vi "Modbus Comm Tester.vi"() -> ()   [LabVIEW 2012]
doc: "Modbus Comm Tester\n\nThis VI demonstrates the usage of the Modbus Master API for both TCP and Serial connections.\nIt is also a useful tool for testing communication with your modbus device. You can test different\ncommunication parameters and coil/register address ranges without having to write any code.\n\nCopyright (c) 2016, Plasmionique Inc.\nAll rights reserved.\n\nLicense: BSD (2-Clause) - http://opensource.org/licenses/BSD-2-Clause"
uses:
  MB_PDU/MB_ReadDevID Codes.ctl
  MB_Master/MB_Master.lvclass
  MB_Master_TCP/MB_Master_TCP.lvclass
  MB_ADU/MB_ADU.lvclass/MB_ADU.ctl
  MB_ADU/Read TX Data.vi
  MB_ADU/Read RX Data.vi
  MB_ADU/Read RX Timestamp.vi
  MB_Master_Serial/MB_Master_Serial.lvclass
  MB Master.lvlib
  MB_ADU/MB_ADU.lvclass
panel:
  in  "Device ID code":T1=1 items=["Basic"=1, "Regular"=2, "Extended"=3, "Single"=4]
  in  "object ID":u8 caption="Object ID"
  in  "Read ID":bool
  out "Open?":bool caption="Connected"
  in  "Tab Control 2":enum32{"Comm Settings", "Comm Status"}(tab)
  in  "Open":bool
  in  "Close":bool
  in  "Type":enum16{"Serial", "TCP"}(ring) caption="Connection Type"
  in  "Tab Control":enum32{"Page 1", "Page 2"}(tab)
  in  "Retries":i32=1
  in  "Timeout (ms)":u32=300
  in  "Flow Control":u16(ring) items=["None", "XON/XOFF", "RTS/CTS", "XON/XOFF & RTS/CTS", "DTR/DSR", "XON/XOFF & DTR/DSR"]
  in  "Parity":u16(ring) items=["None", "Odd", "Even", "Mark", "Space"]
  in  "Stop Bits":u16(ring)=10 items=["1.0"=10, "1.5"=15, "2.0"=20]
  in  "Baud Rate (bps)":u32(ring)=19200 items=["9600"=9600, "19200"=19200, "38400"=38400, "57600"=57600, "115200"=115200, "460800"=460800, "921600"=921600]
  in  "Slave Address":u8=1
  in  "Mode":enum16{"RTU", "ASCII"}(ring)
  in  "COM Port":refnum<visa-resource-name>
  in  "TCP_Port":u16=502 caption="Port"
  in  "IP Address":string="localhost"
  in  "TCP_Timeout":i32=10000 caption="Timeout (ms)"
  in  "TCP_Slave ID":u8=255 caption="Slave ID" format="%.0x"
  in  "Poll Period (ms)":i32=100
  out "Last Error Status":errorcluster
  out "Last RX":string
  out "Last TX":string
  out "Last RX Time":string
  out "Last Error Time":string
  out "dt (ms)":u32
  out "ID objects":string[](array[string]) caption="ID Objects"
  in  "coil Poll":bool
  in  "HR Poll":bool
  in  "DI Poll":bool
  in  "IR Poll":bool
  in  "Write Hld Regs":bool
  in  "Read Hld Regs":bool
  in  "HR QTY":u16=1 caption="Quantity"
  in  "HR SA":u16 caption="Starting Address" format="%.0x"
  in  "Holding Registers":u16[](array[numeric])
  in  "Read In Regs":bool
  in  "IR QTY":u16=1 caption="Quantity"
  in  "IR SA":u16 caption="Starting Address" format="%.0x"
  out "Input Registers":u16[](array[numeric])
  in  "Read DIs":bool
  in  "DI QTY":u16=1 caption="Quantity"
  in  "DI SA":u16 caption="Starting Address" format="%.0x"
  out "Discrete Inputs":bool[](array[boolean])
  in  "Write Coils":bool
  in  "Read Coils":bool
  in  "Coil QTY":u16=1 caption="Quantity"
  in  "Coil SA":u16 caption="Starting Address" format="%.0x"
  in  "Coils":bool[](array[boolean])
  # "Input Registers"
  # "Discrete Inputs"
  # "Device ID Objects"
  # "Holding Registers"
  # "Coils"
  # "Communication Settngs"
  # "Communication Status"
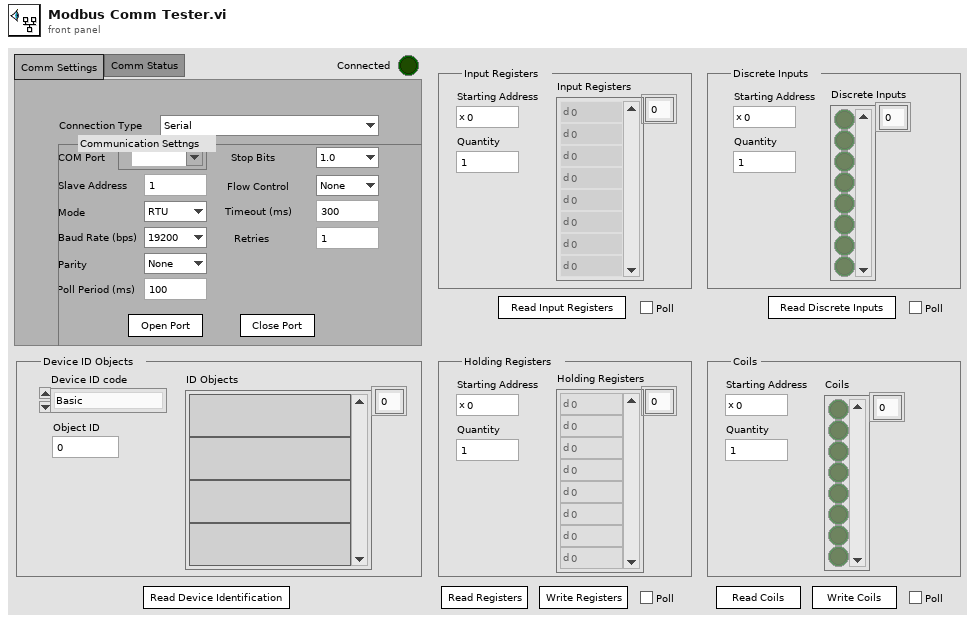
[diagram p1: front panel]
types:
  T1 = typedef "MB Master.lvlib/MB_ReadDevID Codes.ctl" = u8
  T2 = cluster{"baud rate (bps)":u32, "stop bits":u16, "parity":u16, "flow control":u16, "timeout":u32, "retries":i32}
  T3 = typedef "MB Master.lvlib/MB_DevID Object.ctl" = cluster{"ID":u8, "Value":string}
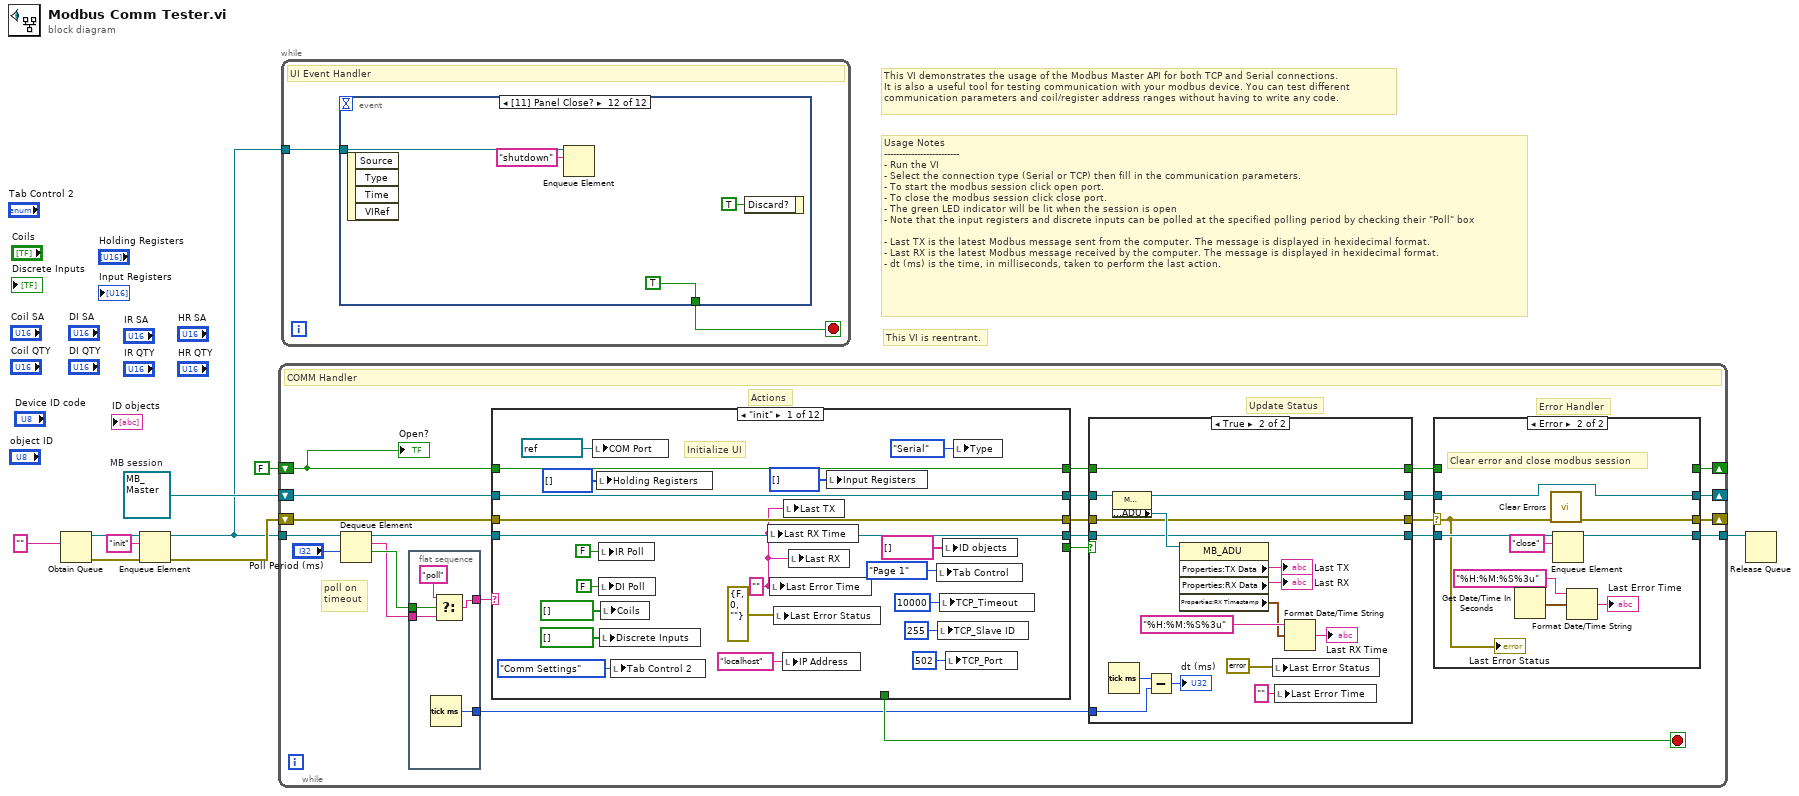
[diagram p0: block diagram]
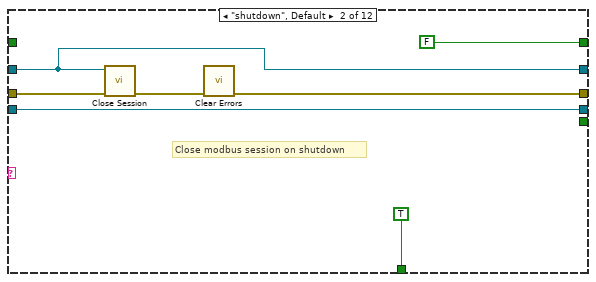
[diagram p4: hidden frame]
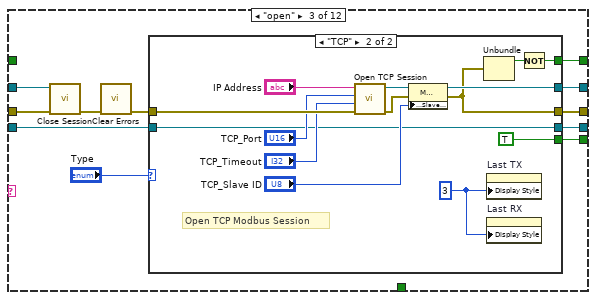
[diagram p5: hidden frame]
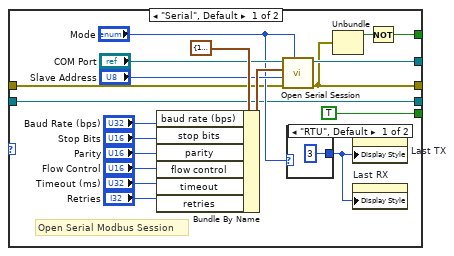
[diagram p6: hidden frame]
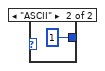
[diagram p7: hidden frame]
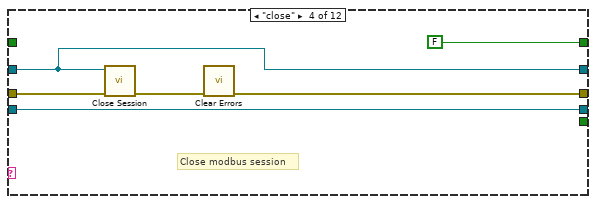
[diagram p8: hidden frame]
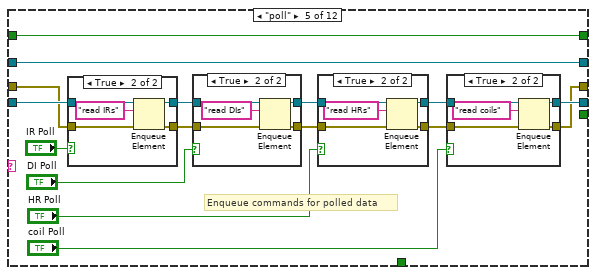
[diagram p9: hidden frame]
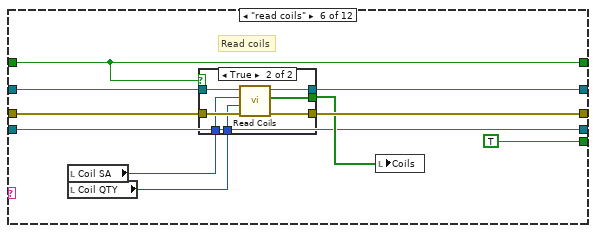
[diagram p14: hidden frame]
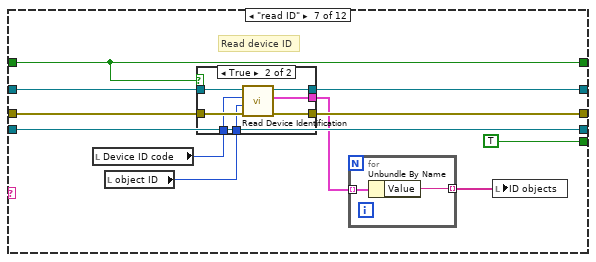
[diagram p16: hidden frame]
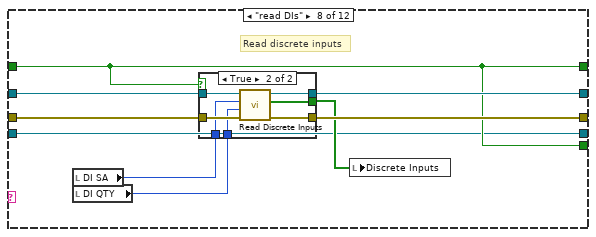
[diagram p18: hidden frame]
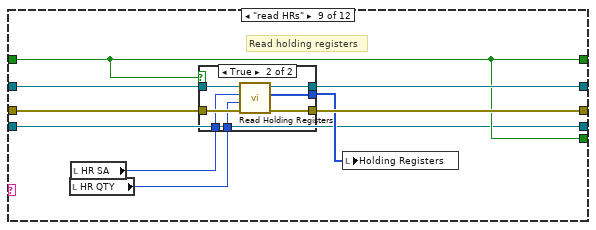
[diagram p20: hidden frame]
diagram:
  w7 = refnum<class "MB_Master.lvclass"> refnum  # MB session
  # "This VI is reentrant."
  # "Usage Notes\n-------------------------\n- Run the VI\n- Select the connection type (Serial or TCP) then fill in the communication parameters.\n- To start the modbus session click open port.\n- To close the modbus session click close port.\n- The green LED indicator will be lit when the session is open\n- Note that the input registers and discrete inputs can be polled at the specified polling period by checking their \"Poll\" box\n\n- Last TX is the latest Modbus message sent from the computer. The message is displayed in hexidecimal format.\n- Last RX is the latest Modbus message received by the computer. The message is displayed in hexidecimal format. \n- dt (ms) is the time, in milliseconds, taken to perform the last action."
  # "This VI demonstrates the usage of the Modbus Master API for both TCP and Serial connections.\nIt is also a useful tool for testing communication with your modbus device. You can test different\ncommunication parameters and coil/register address ranges without having to write any code."
  n1 = Obtain Queue(element data type="") -> (queue out=w6:refnum<queue>, error out=w4:errorcluster)  [unwired: 4 in, 1 out]
  n2 = Enqueue Element(queue=w6, element="init", error in (no error)=w4) -> (queue out=w2:refnum<queue>, error out=w3:errorcluster)  [unwired: 1 in, 1 out]
  n3 = while {
    tunnel: w2 -> [w33]
    shift-right: [w16] -> _
    shift-left: w7 -> [w32]
    shift-right: [w23] -> _
    shift-left: w3 -> [w24]
    shift-right: [w18] -> _
    shift-left: FALSE -> [w28]
    tunnel: [w22] -> w1
    stop <- w31 stop-if-true
    # "poll on\ntimeout"
    # "Actions"
    # "Error Handler"
    # "Update Status"
    # "COMM Handler"
    n4 = Dequeue Element(queue=w33, timeout in ms (-1)="Poll Period (ms)") -> (queue out=w30:refnum<queue>, element=w20:string, timed out?=w21:bool)  [unwired: 1 in, 1 out]
    n5 = flat-sequence {
      tunnel: [w51] -> w25
      tunnel: w21 -> [w50]
      tunnel: w20 -> [w49]
      tunnel: [w47] -> w19
      frame #0 {
        n6 = Tick Count (ms)() -> (millisecond timer value=w51:u32)
        n7 = Select(t="poll", s=w50, f=w49) -> (s? t:f=w47:string)
      }
    }
    n8 = case shown="\"init\"" w19 {
      tunnel: [w91 w96 w110 w148 w160 w203 w223 w243 w261 w279 w299 w333] -> w29
      tunnel: w32 -> [w91 w96 w105 w148 w160 w205 w225 w245 w263 w281 w302 w336]
      tunnel: [w90 w97 w109 w149 w152 w202 w222 w242 w260 w278 w297 w331] -> w13
      tunnel: w24 -> [w90 w99 w104 w151 w164 w204 w224 w244 w262 w280 w298 w332]
      tunnel: [_ TRUE _ _ _ _ _ _ _ _ _ _] -> w31
      tunnel: w30 -> [w81 w93 w101 w146 w166 w196 w219 w237 w255 w273 w291 w325]
      tunnel: w28 -> [w88 _ _ _ w161 w200 w221 w238 w256 w274 w292 w326]
      tunnel: [w88 FALSE w108 FALSE w161 w200 w221 w238 w256 w274 w292 w326] -> w15
      tunnel: [_ _ w107 _ _ TRUE TRUE w238 w256 w274 w292 w326] -> w27
      tunnel: [w81 w93 w100 w146 w158 w196 w219 w237 w255 w273 w291 w325] -> w11
      frame "init" {
        w89 = "" ("Last Error Time")
        # "Initialize UI"
        n9 = local write "COM Port"(refnum<visa-resource-name> refnum ("COM Port")) -> ()
        n10 = local write "Holding Registers"(u16[] [] ("Holding Registers")) -> ()
        n11 = local write "IR Poll"(FALSE ("IR Poll")) -> ()
        n12 = local write "DI Poll"(FALSE ("DI Poll")) -> ()
        n13 = local write "Discrete Inputs"(bool[] [] ("Coils")) -> ()
        n14 = local write "Coils"(bool[] [] ("Coils")) -> ()
        n15 = local write "Tab Control 2"(enum32{"Comm Settings", "Comm Status"}."Comm Settings" ("Tab Control 2")) -> ()
        n16 = local write "Last RX Time"(w89) -> ()
        n17 = local write "Last Error Time"(w89) -> ()
        n18 = local write "Last Error Status"(errorcluster {"status"=FALSE, "code"=0, "source"=""} ("Last Error Status")) -> ()
        n19 = local write "IP Address"("localhost" ("IP Address")) -> ()
        n20 = local write "Last TX"(w89) -> ()
        n21 = local write "Last RX"(w89) -> ()
        n22 = local write "Input Registers"(u16[] [] ("Input Registers")) -> ()
        n23 = local write "Tab Control"(enum32{"Page 1", "Page 2"}."Page 1" ("Tab Control")) -> ()
        n24 = local write "TCP_Slave ID"(u8 255 ("TCP_Slave ID")) -> ()
        n25 = local write "TCP_Timeout"(10000 ("TCP_Timeout")) -> ()
        n26 = local write "ID objects"(string[] [] ("ID objects")) -> ()
        n27 = local write "TCP_Port"(u16 502 ("TCP_Port")) -> ()
        n28 = local write "Type"(enum16{"Serial", "TCP"}."Serial" ("Type")) -> ()
      }
      frame "shutdown", Default {
        # "Close modbus session on shutdown"
        n29 = call-dynamic "Close Session.vi"("error in (no error)"=w99, "MB session in"=w96) -> ("error out"=w98:errorcluster)  [unwired: 9 in]
        n30 = call <vilib>:"Clear Errors.vi"("error in (no error)"=w98) -> ("error out"=w97:errorcluster)  [unwired: 6 in]
      }
      frame "open" {
        n31 = call-dynamic "Close Session.vi"("error in (no error)"=w104, "MB session in"=w105) -> ("error out"=w106:errorcluster)  [unwired: 9 in]
        n32 = call <vilib>:"Clear Errors.vi"("error in (no error)"=w106) -> ("error out"=w103:errorcluster)  [unwired: 6 in]
        n33 = case shown="\"TCP\"" "Type" {
          tunnel: [w119 w136] -> w110
          tunnel: [w118 w134] -> w109
          tunnel: [w116 w133] -> w108
          tunnel: [TRUE TRUE] -> w107
          tunnel: w103 -> [w112 w143]
          tunnel: [w111 w137] -> w100
          tunnel: w101 -> [w111 w137]
          frame "Serial", Default {
            # "Open Serial Modbus Session"
            n34 = Bundle By Name(cluster=T2 {"baud rate (bps)"=19200, "stop bits"=10, "parity"=0, "flow control"=0, "timeout"=1000, "retries"=1} ("Serial Config"), "baud rate (bps)"="Baud Rate (bps)", "stop bits"="Stop Bits", "parity"="Parity", "flow control"="Flow Control", "timeout"="Timeout (ms)", "retries"="Retries") -> (w121:T2)
            n35 = call "Open Serial Session.vi"("Mode (RTU)"="Mode", "Error in"=w112, "Slave ID"="Slave Address", "Serial Config"=w121, "VISA Resource"="COM Port") -> ("Error out"=w118:errorcluster, "MB_Serial session"=w119:refnum<class "MB_Master_Serial.lvclass">)  [unwired: 5 in]
            n36 = case shown="\"RTU\", Default" "Mode" {
              tunnel: [u32 3 ("Display Style") u32 1 ("Display Style")] -> w113
              frame "RTU", Default {
              }
              frame "ASCII" {
              }
            }
            n37 = Unbundle(w118) -> ("status"=w117:bool)  [unwired: 2 out]
            n38 = property on="Last TX" class="Str"("Display Style"=w113) -> ()  [unwired: 2 in, 2 out]
            n39 = property on="Last RX" class="Str"("Display Style"=w113) -> ()  [unwired: 2 in, 2 out]
            n40 = Not(x=w117) -> (.not. x?=w116:bool)
          }
          frame "TCP" {
            w132 = u32 3 ("Display Style")
            # "Open TCP Modbus Session"
            n41 = call "Open TCP Session.vi"("error in (no error)"=w143, "Timeout (10000)"="TCP_Timeout", "Port (502)"="TCP_Port", "IP Address"="IP Address") -> ("error out"=w144:errorcluster, "MB_TCP session"=w145:refnum<class "MB_Master_TCP.lvclass">)  [unwired: 6 in]
            n42 = property class="MB_Master_TCP"(reference=w145, error in=w144, "Properties:Slave ID"="TCP_Slave ID") -> (reference out=w136:refnum<class "MB_Master_TCP.lvclass">, error out=w134:errorcluster)
            n43 = Unbundle(w134) -> ("status"=w135:bool)  [unwired: 2 out]
            n44 = property on="Last TX" class="Str"("Display Style"=w132) -> ()  [unwired: 2 in, 2 out]
            n45 = property on="Last RX" class="Str"("Display Style"=w132) -> ()  [unwired: 2 in, 2 out]
            n46 = Not(x=w135) -> (.not. x?=w133:bool)
          }
        }
      }
      frame "close" {
        # "Close modbus session"
        n47 = call-dynamic "Close Session.vi"("error in (no error)"=w151, "MB session in"=w148) -> ("error out"=w150:errorcluster)  [unwired: 9 in]
        n48 = call <vilib>:"Clear Errors.vi"("error in (no error)"=w150) -> ("error out"=w149:errorcluster)  [unwired: 6 in]
      }
      frame "poll" {
        # "Enqueue commands for polled data"
        n49 = case shown="True" "IR Poll" {
          tunnel: w166 -> [w190 w194]
          tunnel: [w190 w193] -> w165
          tunnel: w164 -> [w189 w192]
          tunnel: [w189 w191] -> w162
          frame False {
          }
          frame True {
            n50 = Enqueue Element(queue=w194, element="read IRs", error in (no error)=w192) -> (queue out=w193:refnum<queue>, error out=w191:errorcluster)  [unwired: 1 in, 1 out]
          }
        }
        n51 = case shown="True" "DI Poll" {
          tunnel: w165 -> [w182 w187]
          tunnel: w162 -> [w183 w186]
          tunnel: [w183 w185] -> w156
          tunnel: [w182 w184] -> w159
          frame False {
          }
          frame True {
            n52 = Enqueue Element(queue=w187, element="read DIs", error in (no error)=w186) -> (queue out=w184:refnum<queue>, error out=w185:errorcluster)  [unwired: 1 in, 1 out]
          }
        }
        n53 = case shown="True" "HR Poll" {
          tunnel: w159 -> [w175 w180]
          tunnel: w156 -> [w176 w179]
          tunnel: [w176 w178] -> w154
          tunnel: [w175 w177] -> w157
          frame False {
          }
          frame True {
            n54 = Enqueue Element(queue=w180, element="read HRs", error in (no error)=w179) -> (queue out=w177:refnum<queue>, error out=w178:errorcluster)  [unwired: 1 in, 1 out]
          }
        }
        n55 = case shown="True" "coil Poll" {
          tunnel: w157 -> [w168 w173]
          tunnel: w154 -> [w169 w172]
          tunnel: [w169 w171] -> w152
          tunnel: [w168 w170] -> w158
          frame False {
          }
          frame True {
            n56 = Enqueue Element(queue=w173, element="read coils", error in (no error)=w172) -> (queue out=w170:refnum<queue>, error out=w171:errorcluster)  [unwired: 1 in, 1 out]
          }
        }
      }
      frame "read coils" {
        # "Read coils"
        n57 = local read "Coil SA"() -> (w199:u16)
        n58 = local read "Coil QTY"() -> (w198:u16)
        n59 = case shown="True" w200 {
          tunnel: w205 -> [w207 w214]
          tunnel: w204 -> [w206 w213]
          tunnel: [w207 w212] -> w203
          tunnel: [w206 w211] -> w202
          tunnel: w199 -> [_ w210]
          tunnel: w198 -> [_ w209]
          tunnel: [_ w208] -> w201
          frame False {
          }
          frame True {
            n60 = call "Read Coils.vi"("error in (no error)"=w213, "quantity"=w209, "starting address"=w210, "MB session in"=w214) -> ("error out"=w211:errorcluster, "Coils"=w208:bool[], "MB session out"=w212:refnum<class "MB_Master.lvclass">)  [unwired: 5 in]
          }
        }
        n61 = local write "Coils"(w201) -> ()
      }
      frame "read ID" {
        # "Read device ID"
        n62 = local read "Device ID code"() -> (w217:T1)
        n63 = local read "object ID"() -> (w218:u8)
        n64 = case shown="True" w221 {
          tunnel: w225 -> [w229 w234]
          tunnel: w224 -> [w228 w236]
          tunnel: [w229 w233] -> w223
          tunnel: [w228 w235] -> w222
          tunnel: [_ w232] -> w216
          tunnel: w218 -> [_ w231]
          tunnel: w217 -> [_ w230]
          frame False {
          }
          frame True {
            n65 = call "Read Device Identification.vi"("error in (no error)"=w236, "object ID"=w231, "read device ID code"=w230, "MB session in"=w234) -> ("error out"=w235:errorcluster, "DevID Objects"=w232:T3[], "MB session out"=w233:refnum<class "MB_Master.lvclass">)  [unwired: 4 in, 1 out]
          }
        }
        n66 = for {
          tunnel: w216 -> [w227] mode=indexing
          tunnel: [w226] -> w215 mode=indexing
          n67 = Unbundle By Name(w227) -> ("Value"=w226:string)
        }
        n68 = local write "ID objects"(w215) -> ()
      }
      frame "read DIs" {
        # "Read discrete inputs"
        n69 = local read "DI SA"() -> (w240:u16)
        n70 = local read "DI QTY"() -> (w239:u16)
        n71 = case shown="True" w238 {
          tunnel: w245 -> [w247 w254]
          tunnel: w244 -> [w246 w253]
          tunnel: [w247 w252] -> w243
          tunnel: [w246 w251] -> w242
          tunnel: w240 -> [_ w250]
          tunnel: w239 -> [_ w249]
          tunnel: [_ w248] -> w241
          frame False {
          }
          frame True {
            n72 = call "Read Discrete Inputs.vi"("error in (no error)"=w253, "quantity"=w249, "starting address"=w250, "MB session in"=w254) -> ("error out"=w251:errorcluster, "Inputs"=w248:bool[], "MB session out"=w252:refnum<class "MB_Master.lvclass">)  [unwired: 5 in]
          }
        }
        n73 = local write "Discrete Inputs"(w241) -> ()
      }
      frame "read HRs" {
        # "Read holding registers"
        n74 = local read "HR QTY"() -> (w257:u16)
        n75 = local read "HR SA"() -> (w258:u16)
        n76 = case shown="True" w256 {
          tunnel: w263 -> [w265 w272]
          tunnel: w262 -> [w264 w271]
          tunnel: [w265 w270] -> w261
          tunnel: [w264 w269] -> w260
          tunnel: w258 -> [_ w268]
          tunnel: w257 -> [_ w267]
          tunnel: [_ w266] -> w259
          frame False {
          }
          frame True {
            n77 = call "Read Holding Registers.vi"("error in (no error)"=w271, "quantity"=w267, "starting address"=w268, "MB session in"=w272) -> ("error out"=w269:errorcluster, "Registers"=w266:u16[], "MB session out"=w270:refnum<class "MB_Master.lvclass">)  [unwired: 5 in]
          }
        }
        n78 = local write "Holding Registers"(w259) -> ()
      }
      frame "read IRs" {
        # "Read input registers"
        n79 = local read "IR QTY"() -> (w275:u16)
        n80 = local read "IR SA"() -> (w276:u16)
        n81 = case shown="True" w274 {
          tunnel: w281 -> [w283 w290]
          tunnel: w280 -> [w282 w289]
          tunnel: [w283 w288] -> w279
          tunnel: [w282 w287] -> w278
          tunnel: w276 -> [_ w286]
          tunnel: w275 -> [_ w285]
          tunnel: [_ w284] -> w277
          frame False {
          }
          frame True {
            n82 = call "Read Input Registers.vi"("error in (no error)"=w289, "quantity"=w285, "starting address"=w286, "MB session in"=w290) -> ("error out"=w287:errorcluster, "Registers"=w284:u16[], "MB session out"=w288:refnum<class "MB_Master.lvclass">)  [unwired: 5 in]
          }
        }
        n83 = local write "Input Registers"(w277) -> ()
      }
      frame "write coils" {
        # "Write single or multiple coils"
        n84 = local read "Coil SA"() -> (w296:u16)
        n85 = local read "Coil QTY"() -> (w294:u16)
        n86 = local read "Coils"() -> (w295:bool[])
        n87 = Greater?(x=w294, y=u16 1) -> (0:w300:bool)
        n88 = Array Subset(array=w295, length=w294) -> (w293:bool[])  [unwired: 1 in]
        n89 = case shown="True" w292 {
          tunnel: w302 -> [w304 w311]
          tunnel: w300 -> [_ w310]
          tunnel: [w304 w309] -> w299
          tunnel: w298 -> [w303 w308]
          tunnel: [w303 w307] -> w297
          tunnel: w296 -> [_ w306]
          tunnel: w293 -> [_ w305]
          frame False {
          }
          frame True {
            n90 = case shown="True" w310 {
              tunnel: w311 -> [w318 w324]
              tunnel: [w312 w323] -> w309
              tunnel: w308 -> [w317 w322]
              tunnel: [w313 w321] -> w307
              tunnel: w306 -> [w316 w320]
              tunnel: w305 -> [w315 w319]
              frame False {
                n91 = Index Array(array=w315) -> (element=w314:bool)  [unwired: 1 in]
                n92 = call "Write Single Coil.vi"("error in (no error)"=w317, "value"=w314, "address"=w316, "MB session in"=w318) -> ("error out"=w313:errorcluster, "MB session out"=w312:refnum<class "MB_Master.lvclass">)  [unwired: 6 in]
              }
              frame True {
                n93 = call "Write Multiple Coils.vi"("error in (no error)"=w322, "values"=w319, "starting address"=w320, "MB session in"=w324) -> ("error out"=w321:errorcluster, "MB session out"=w323:refnum<class "MB_Master.lvclass">)  [unwired: 6 in]
              }
            }
          }
        }
      }
      frame "write HRs" {
        # "Write single or multiple holding registers"
        n94 = local read "Holding Registers"() -> (w329:u16[])
        n95 = local read "HR QTY"() -> (w328:u16)
        n96 = local read "HR SA"() -> (w330:u16)
        n97 = Greater?(x=w328, y=u16 1) -> (0:w334:bool)
        n98 = Array Subset(array=w329, length=w328) -> (w327:u16[])  [unwired: 1 in]
        n99 = case shown="True" w326 {
          tunnel: w336 -> [w338 w345]
          tunnel: w334 -> [_ w344]
          tunnel: [w338 w343] -> w333
          tunnel: w332 -> [w337 w342]
          tunnel: [w337 w341] -> w331
          tunnel: w330 -> [_ w340]
          tunnel: w327 -> [_ w339]
          frame False {
          }
          frame True {
            n100 = case shown="True" w344 {
              tunnel: w345 -> [w352 w358]
              tunnel: [w346 w357] -> w343
              tunnel: w342 -> [w351 w356]
              tunnel: [w347 w355] -> w341
              tunnel: w340 -> [w350 w354]
              tunnel: w339 -> [w349 w353]
              frame False {
                n101 = Index Array(array=w349) -> (element=w348:u16)  [unwired: 1 in]
                n102 = call "Write Single Register.vi"("error in (no error)"=w351, "value"=w348, "address"=w350, "MB session in"=w352) -> ("error out"=w347:errorcluster, "MB session out"=w346:refnum<class "MB_Master.lvclass">)  [unwired: 6 in]
              }
              frame True {
                n103 = call "Write Multiple Registers.vi"("error in (no error)"=w356, "values"=w353, "starting address"=w354, "MB session in"=w358) -> ("error out"=w355:errorcluster, "MB session out"=w357:refnum<class "MB_Master.lvclass">)  [unwired: 6 in]
              }
            }
          }
        }
      }
    }
    n104 = case shown="True" w27 {
      tunnel: w29 -> [w55 w56]
      tunnel: [w55 w69] -> w17
      tunnel: w25 -> [_ w63]
      tunnel: w15 -> [w54 w59]
      tunnel: [w54 w59] -> w14
      tunnel: w13 -> [w53 w58]
      tunnel: [w53 w58] -> w12
      tunnel: w11 -> [w52 w57]
      tunnel: [w52 w57] -> w10
      frame False {
      }
      frame True {
        n105 = Tick Count (ms)() -> (millisecond timer value=w62:u32)
        n106 = property class="MB_Master"(reference=w56) -> (reference out=w69:refnum<class "MB_Master.lvclass">, "Properties:ADU"=w70:refnum<class "MB_ADU.lvclass">)  [unwired: 1 in, 1 out]
        n107 = Subtract(x=w62, y=w63) -> (x-y=→"dt (ms)":u32)
        n108 = property class="MB_ADU"(reference=w70) -> ("Properties:TX Data"=→"Last TX":string, "Properties:RX Data"=→"Last RX":string, "Properties:RX Timestamp"=w60:timestamp)  [unwired: 1 in, 2 out]
        n109 = local write "Last Error Status"(errorcluster {"status"=FALSE, "code"=0, "source"=""} ("Last Error Status")) -> ()
        n110 = local write "Last Error Time"("" ("Last Error Time")) -> ()
        n111 = Format Date/Time String(time format string (%c)="%H:%M:%S%3u", seconds (now)=w60) -> (date/time string=→"Last RX Time":string)  [unwired: 1 in]
      }
    }
    n112 = case shown="Error" w12 {
      selector: w12 -> [w37 w39]
      tunnel: [w37 w43] -> w23
      tunnel: w10 -> [w36 w41]
      tunnel: [w36 w40] -> w22
      tunnel: w14 -> [w35 _]
      tunnel: [w35 _] -> w18
      tunnel: w17 -> [w34 w38]
      tunnel: [w34 w38] -> w16
      frame No Error {
      }
      frame Error {
        # "Clear error and close modbus session"
        n113 = Get Date/Time In Seconds() -> (seconds since 1Jan1904=w44:timestamp)
        n114 = call <vilib>:"Clear Errors.vi"("error in (no error)"=w39) -> ("error out"=w43:errorcluster)  [unwired: 6 in]
        n115 = Enqueue Element(queue=w41, element="close") -> (queue out=w40:refnum<queue>)  [unwired: 2 in, 2 out]
        n116 = Format Date/Time String(time format string (%c)="%H:%M:%S%3u", seconds (now)=w44) -> (date/time string=→"Last Error Time":string)  [unwired: 1 in]
        "Last Error Status" <- w39
      }
    }
    "Open?" <- w28
  }
  n117 = while {
    tunnel: w2 -> [w360]
    stop <- w359 stop-if-true
    # "UI Event Handler"
    n118 = event shown="[11] Panel Close?" {
      selector: _ -> [_ _ _ _ _ _ _ _ _ _ _ _]
      dyn-events: _ -> [_ _ _ _ _ _ _ _ _ _ _ _]
      timeout: _ -> [_ _ _ _ _ _ _ _ _ _ _ _]
      tunnel: w360 -> [_ w364 w367 w368 w370 w372 w374 w376 w378 w380 w382 w384]
      tunnel: [_ _ _ _ _ _ _ _ _ _ _ TRUE] -> w359
      event Timeout {
        n119 = event-data() -> ()  [unwired: 1 in, 3 out]
      }
      event "Type": Value Change {
        # "Transparent (invisible) tab control contains comm parameter controls"
        # "Change connection type"
        n120 = event-data() -> ("NewVal"=w363:enum16{"Serial", "TCP"})  [unwired: 1 in, 5 out]
        n121 = Type Cast(type="Tab Control", x=w363) -> (*(type *) &x=w361:enum32{"Page 1", "Page 2"})
        n122 = local write "Tab Control"(w361) -> ()
        n123 = Enqueue Element(queue=w364, element="close") -> ()  [unwired: 2 in, 3 out]
      }
      event "Open": Value Change {
        # "Open modbus session"
        n124 = event-data() -> ()  [unwired: 1 in, 6 out]
        n125 = Enqueue Element(queue=w367, element="open") -> ()  [unwired: 2 in, 3 out]
      }
      event "Close": Value Change {
        # "Close modbus session"
        n126 = event-data() -> ()  [unwired: 1 in, 6 out]
        n127 = Enqueue Element(queue=w368, element="close") -> ()  [unwired: 2 in, 3 out]
      }
      event "Read Coils": Value Change {
        n128 = event-data() -> ()  [unwired: 1 in, 6 out]
        n129 = Enqueue Element(queue=w370, element="read coils") -> ()  [unwired: 2 in, 3 out]
      }
      event "Read ID": Value Change {
        n130 = event-data() -> ()  [unwired: 1 in, 6 out]
        n131 = Enqueue Element(queue=w372, element="read ID") -> ()  [unwired: 2 in, 3 out]
      }
      event "Read DIs": Value Change {
        n132 = event-data() -> ()  [unwired: 1 in, 6 out]
        n133 = Enqueue Element(queue=w374, element="read DIs") -> ()  [unwired: 2 in, 3 out]
      }
      event "Write Coils": Value Change {
        n134 = event-data() -> ()  [unwired: 1 in, 6 out]
        n135 = Enqueue Element(queue=w376, element="write coils") -> ()  [unwired: 2 in, 3 out]
      }
      event "Read In Regs": Value Change {
        n136 = event-data() -> ()  [unwired: 1 in, 6 out]
        n137 = Enqueue Element(queue=w378, element="read IRs") -> ()  [unwired: 2 in, 3 out]
      }
      event "Read Hld Regs": Value Change {
        n138 = event-data() -> ()  [unwired: 1 in, 6 out]
        n139 = Enqueue Element(queue=w380, element="read HRs") -> ()  [unwired: 2 in, 3 out]
      }
      event "Write Hld Regs": Value Change {
        n140 = event-data() -> ()  [unwired: 1 in, 6 out]
        n141 = Enqueue Element(queue=w382, element="write HRs") -> ()  [unwired: 2 in, 3 out]
      }
      event Panel Close? {
        n142 = event-data() -> ()  [unwired: 1 in, 4 out]
        n143 = Enqueue Element(queue=w384, element="shutdown") -> ()  [unwired: 2 in, 3 out]
        n144 = event-data("Discard?"=TRUE) -> ()  [unwired: 1 in, 1 out]
      }
    }
  }
  n145 = Release Queue(queue=w1) -> ()  [unwired: 2 in, 3 out]
